vi "Inercia_wheelpendulum.vi"() -> ()   [LabVIEW 2020]
uses:
  <vilib>/addons/control/pid/pid.llb/PID Gain Unit.ctl
  <vilib>/addons/control/pid/pid.llb/PID Structure.ctl
  <vilib>/addons/control/pid/pid.llb/PID Time Unit.ctl
  <vilib>/MakerHub/LINX/Public/Peripherals/Analog/Analog Read 1 Chan.vi
  <vilib>/MakerHub/LINX/Public/Peripherals/Analog/Analog Read N Chans.vi
  <vilib>/MakerHub/LINX/Private/Local IO/LinxAnalogRead.vi
  <vilib>/MakerHub/LINX/Public/Utilities/Check Channel.vi
  <vilib>/MakerHub/LINX/Public/Utilities/Open Serial.vi
  <vilib>/MakerHub/LINX/Private/Utilties/Generate Error.vi
  <vilib>/addons/control/pid/pid.llb/PID Structure Conversion (DBL).vi
  <vilib>/addons/control/pid/pid.llb/PID (DBL).vi
  <vilib>/Analysis/Matrix/Numeric/Conversions/Matrix To Array - RM.vi
  <vilib>/MakerHub/LINX/Public/Peripherals/PWM/PWM Set Duty Cycle N Chans.vi
  <vilib>/MakerHub/LINX/LMH-LINX.lvlib
  <vilib>/Analysis/Matrix/NI_Matrix.lvlib
  <vilib>/addons/control/pid/NI_PID_pid.lvlib
panel:
  out "vitesse commande_2":dbl(graph)
  out "vitesse commande_1":dbl(graph)
  in  "reinitialize? (F) 2":bool
  in  "dt (s) 2":dbl=-1.0 format="%.3f"
  in  "setpoint 2":dbl format="%.2f"
  in  "output range":cluster{"output high":dbl, "output low":dbl}={"output high"=100.0, "output low"=-100.0} {"output low" format="%.2f"; "output high" format="%.2f"}
  in  "derivative unit":T1 items=["min", "s"]
  in  "integral unit":T1 items=["min", "s"]
  in  "PID structure":T2 items=["Academic (Standard)", "Parallel", "Series"]
  in  "proportional unit":T3 items=["Gain (K)", "Band (PB)"]
  in  "derivative":dbl
  in  "integral":dbl
  in  "proportional":dbl
  out "pid":dbl format="%.2f"
  out "dt out (s)":dbl format="%.3f"
  out "angle":dbl(graph)
  out "output angle":dbl
  in  "setpoint":dbl format="%.2f"
  in  "PotentionmM":u8
  out "potentiometer voltage":dbl(graph)
  out "Numeric":dbl
  in  "stop":bool
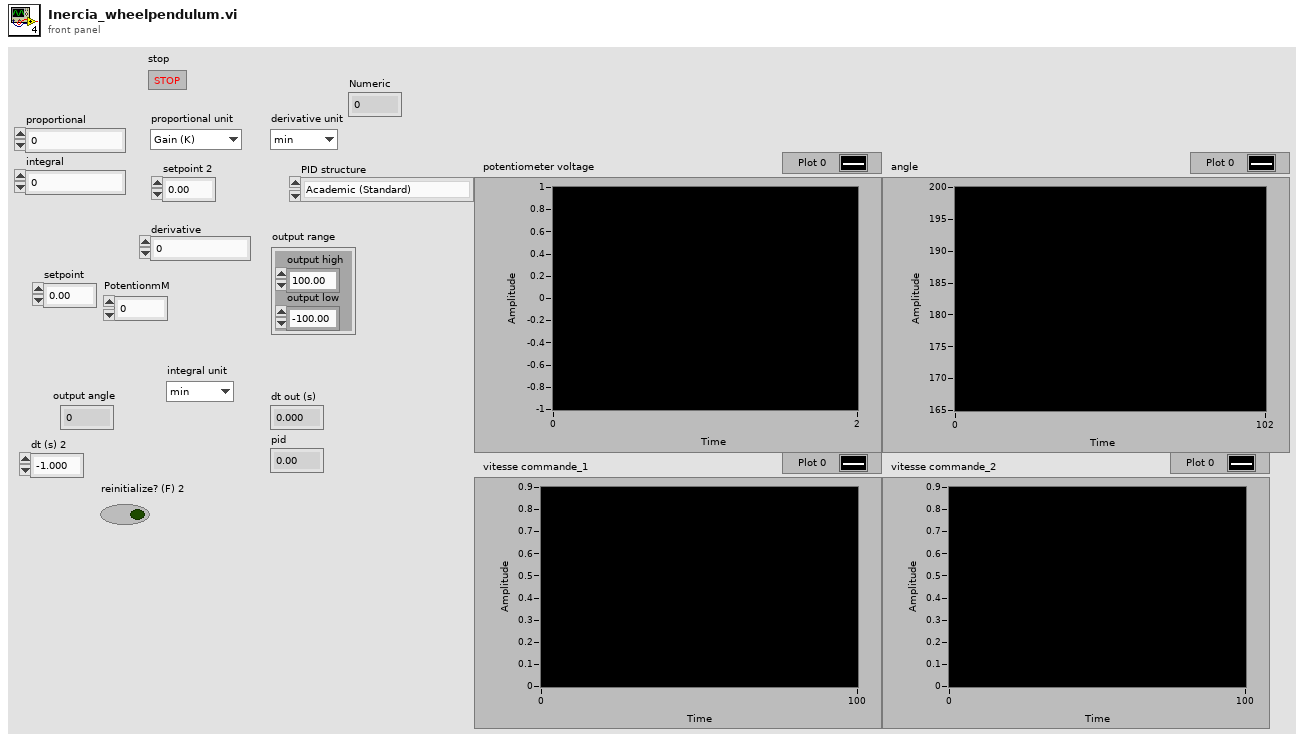
[diagram p1: front panel]
types:
  T1 = typedef "NI_PID_pid.lvlib/PID Time Unit.ctl" = u16
  T2 = typedef "NI_PID_pid.lvlib/PID Structure.ctl" = u16
  T3 = typedef "NI_PID_pid.lvlib/PID Gain Unit.ctl" = u16
  T4 = typedef "LMH-LINX.lvlib/LINX Ref.ctl" = cluster{"IO":T5, "Interface":T6, "LINX Device Config":T7}
  T5 = typedef "LMH-LINX.lvlib/Platform.ctl" = enum16{"Remote", "Local"}
  T6 = typedef "LMH-LINX.lvlib/Interface.ctl" = enum16{"Serial", "TCP"}
  T7 = typedef "LMH-LINX.lvlib/Device.lvlib/LINX Device Config.ctl" = cluster{"Interface":T6, "COM Port":refnum<visa-resource-name>, "TCP Configuration":T8, "Device Family":u8, "Device ID":u8, "Device Name":string, "TCP Ref":refnum<k5>, "Channels":T9}
  T8 = typedef "LMH-LINX.lvlib/Device.lvlib/TCP Config.ctl" = cluster{"IP Address":string, "Port":u16}
  T9 = typedef "LMH-LINX.lvlib/Channels.ctl" = cluster{"DI":u8[], "DO":u8[], "AI":u8[], "AO":u8[], "PWM":u8[], "QE":u8[], "UART":u8[], "I2C 2":u8[], "SPI":u8[], "CAN":u8[], "Servo":u8[], "AI Ref (V)":dbl, "AI Resolution (Bits)":u8, "AO Ref (V)":dbl, "AO Resolution (Bits)":u8}
  T10 = cluster{"proportional gain (Kc)":dbl, "integral time (Ti, min)":dbl, "derivative time (Td, min)":dbl}
  T11 = typedef "NI_Matrix.lvlib/RealMatrix.ctl" = dbl[][]
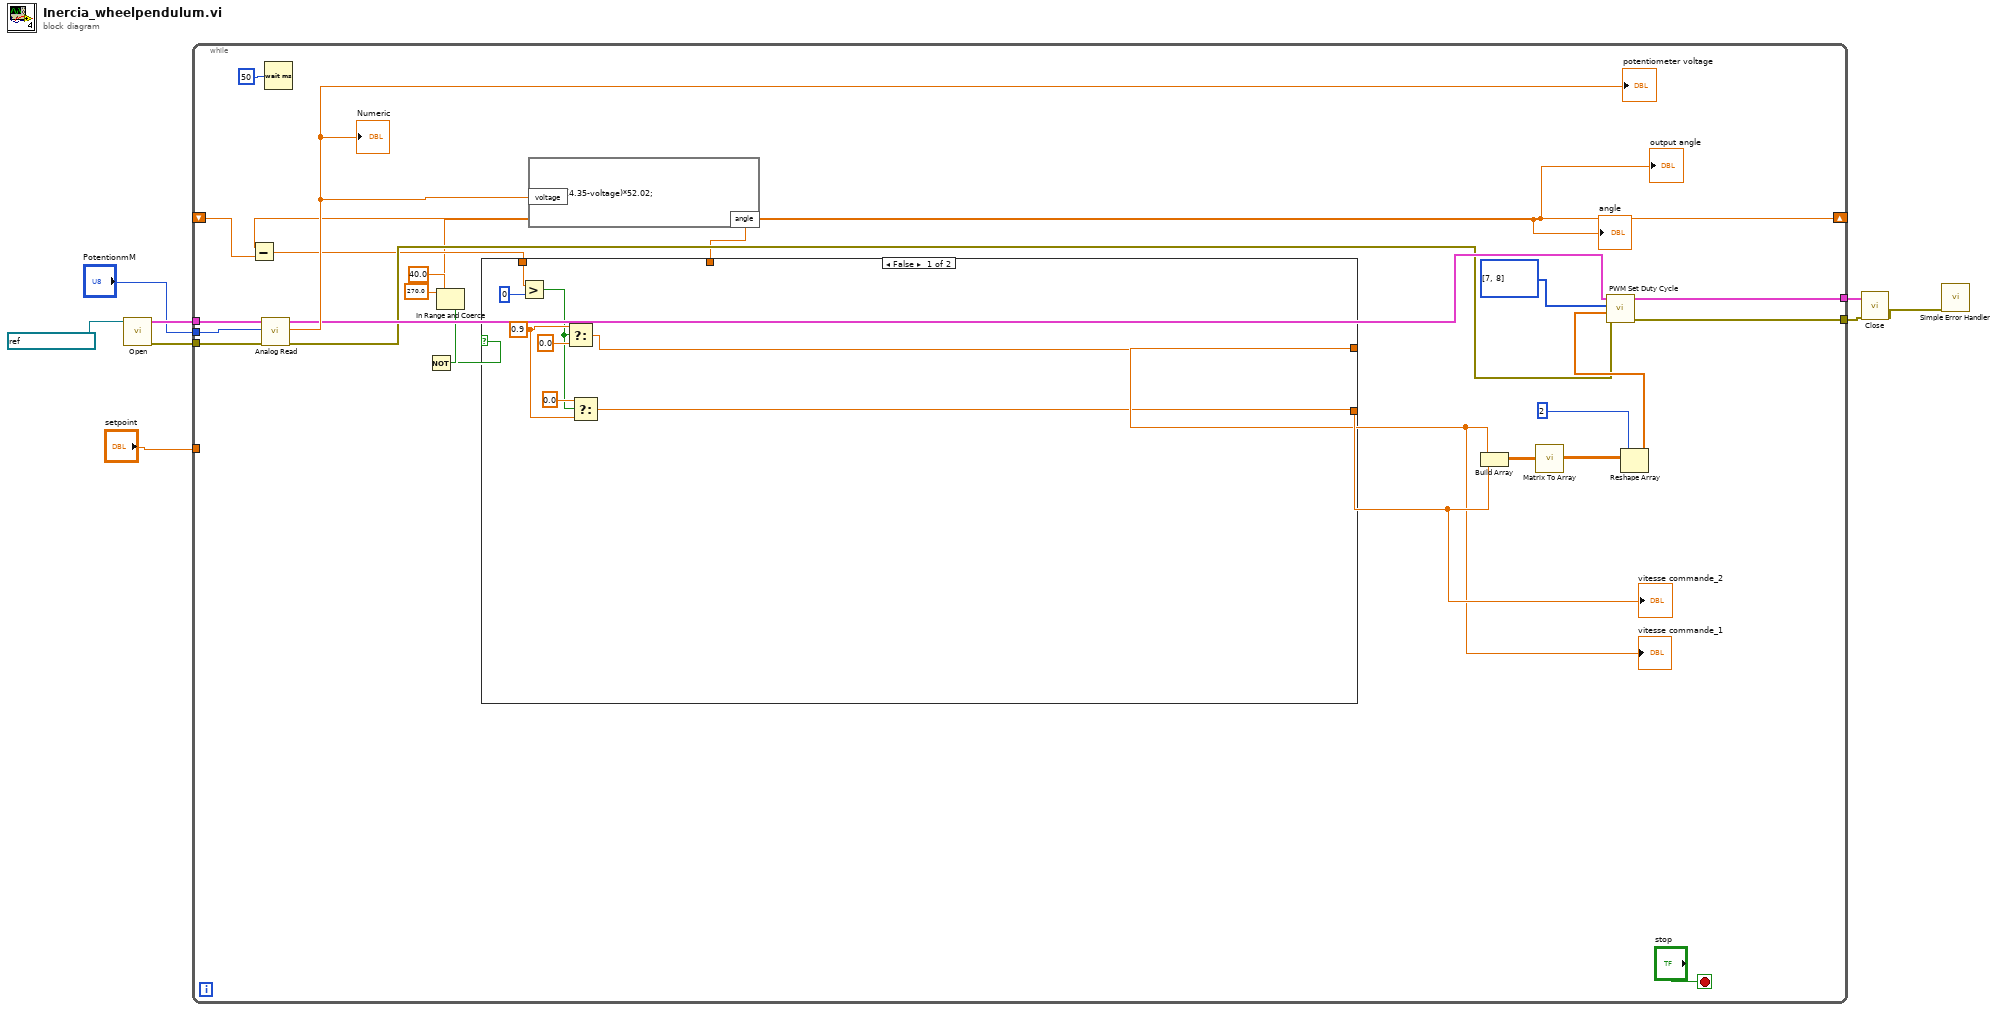
[diagram p0: block diagram]
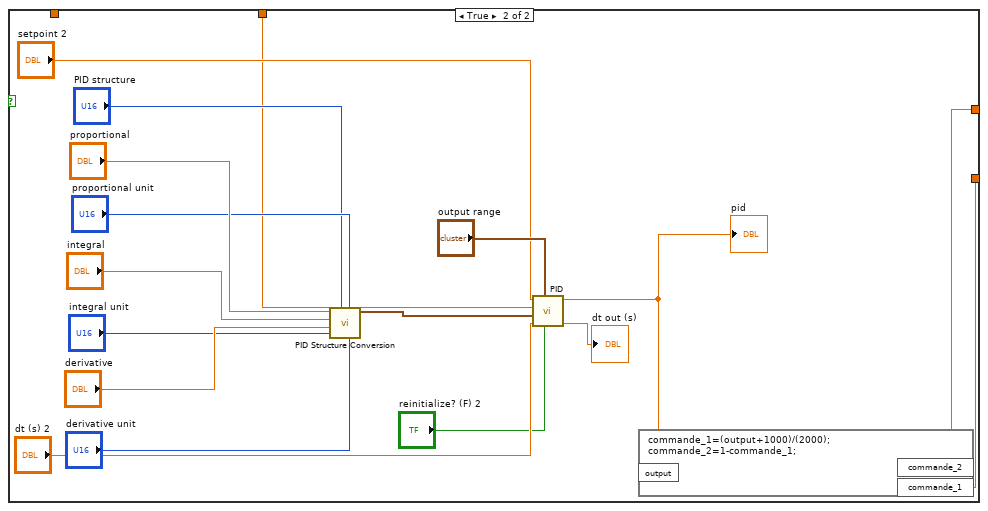
[diagram p2: hidden frame]
diagram:
  n1 = call-poly <vilib>:"Open.vi"("Serial Port"=refnum<visa-resource-name> "ASRL6::INSTR") -> ("Error Out"=w6:errorcluster, "LINX Resource"=w7:T4)  [unwired: 8 in, 1 out]
  n2 = while {
    tunnel: w7 -> [w29]
    tunnel: w6 -> [w28]
    tunnel: "PotentionmM" -> [w31]
    tunnel: "setpoint" -> [_]
    tunnel: [w19] -> w2
    tunnel: [w18] -> w1
    shift-right: [w11] -> _
    shift-left: _ -> [w13]
    stop <- "stop" stop-if-true
    n3 = call-poly <vilib>:"Analog Read.vi"("Error In"=w28, "Analog Channel"=w31, "LINX Resource"=w29) -> ("Error Out"=w20:errorcluster, "Voltage"=w27:dbl, "LINX Resource"=w21:T4)  [unwired: 5 in, 1 out]
    "Numeric" <- w27
    "potentiometer voltage" <- w27
    n4 = Wait (ms)(milliseconds to wait=u32 50) -> ()  [unwired: 1 out]
    n5 = formula code="angle=(4.35-voltage)*52.02;"("voltage"=w27) -> ("angle"=w11:dbl)
    "output angle" <- w11
    "angle" <- w11
    n6 = Subtract(x=w11, y=w13) -> (x-y=w12:dbl)
    n7 = In Range and Coerce(upper limit=270.0, x=w11, lower limit=40.0) -> (In Range?=w15:bool)  [unwired: 1 out]
    n8 = Not(x=w15) -> (.not. x?=w14:bool)
    n9 = case shown="False" w14 {
      tunnel: [w36 w41] -> w10
      tunnel: [w37 w42] -> w9
      tunnel: w12 -> [w33 _]
      tunnel: w11 -> [_ w47]
      frame False {
        w40 = 0.9
        n10 = Greater?(x=w33, y=i16 0) -> (0:w34:bool)
        n11 = Select(t=w40, s=w34, f=0.0) -> (s? t:f=w37:dbl)
        n12 = Select(t=0.0, s=w34, f=w40) -> (s? t:f=w36:dbl)
      }
      frame True {
        n13 = call-poly <vilib>:"PID Structure Conversion.vi"("derivative unit"="derivative unit", "proportional unit"="proportional unit", "integral unit"="integral unit", "PID structure"="PID structure", "derivative"="derivative", "integral"="integral", "proportional"="proportional") -> ("PID gains"=w50:T10)  [unwired: 4 in]
        n14 = call-poly <vilib>:"PID.vi"("reinitialize? (F)"="reinitialize? (F) 2", "output range"="output range", "dt (s)"="dt (s) 2", "PID gains"=w50, "process variable"=w47, "setpoint"="setpoint 2") -> ("dt out (s)"=→"dt out (s)":dbl, "output"=w44:dbl)  [unwired: 4 in]
        "pid" <- w44
        n15 = formula code="commande_1=(output+1000)/(2000);\ncommande_2=1-commande_1;"("output"=w44) -> ("commande_1"=w41:dbl, "commande_2"=w42:dbl)
      }
    }
    "vitesse commande_2" <- w10
    "vitesse commande_1" <- w9
    n16 = Build Array(w9, w10) -> (w24:T11)
    n17 = call-poly <vilib>:"Matrix To Array.vi"("Real Matrix"=w24) -> ("Real 2D Array"=w25:dbl[][])
    n18 = Reshape Array(w25, 2 ("dimension size")) -> (w22:dbl[])
    n19 = call-poly <vilib>:"PWM Set Duty Cycle.vi"("Error In"=w20, "Duty Cycles"=w22, "PWM Channels"=u8[] [7, 8], "LINX Resource"=w21) -> ("Error Out"=w18:errorcluster, "LINX Resource"=w19:T4)  [unwired: 6 in]
  }
  n20 = call <vilib>:"Close.vi"("Error In"=w1, "LINX Resource"=w2) -> ("Error Out"=w5:errorcluster)  [unwired: 9 in]
  n21 = call <vilib>:"Simple Error Handler.vi"("error in (no error)"=w5) -> ()  [unwired: 4 in, 5 out]
